vi "tag bus to outputs.vi"(9 "indices":T1, 11 "tag bus in":T3) -> (2 "data cluster":T2, 3 "tag bus out":T3)   [LabVIEW 2017, in "ActiveFrontEndModule runtime.lvclass"]
uses:
  ActiveFrontEndModule runtime.lvclass
  <vilib>/NI/Tag Bus/table/data table.ctl
  output user data.ctl
  configuration/output data indices.ctl
  <vilib>/NI/Tag Bus/table/data polymorphs/read one/read I32.vi
  <vilib>/NI/Tag Bus/table/data table.lvlib
  configuration/ActiveFrontEndModule configuration.lvclass
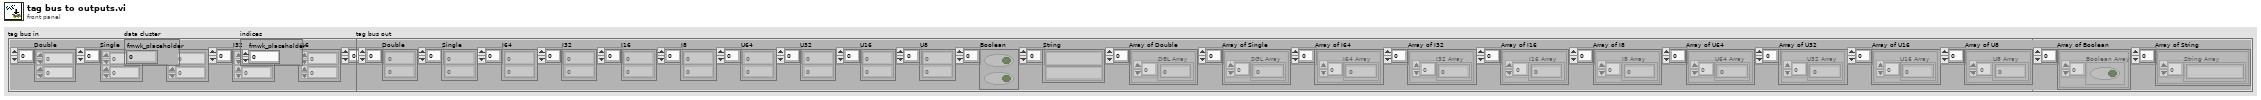
[diagram p1: front panel]
types:
  T1 = typedef "ActiveFrontEndModule configuration.lvclass/output data indices.ctl" = cluster{"fmwk_placeholder":i32}
  T2 = typedef "ActiveFrontEndModule runtime.lvclass/output user data.ctl" = cluster{"fmwk_placeholder":i32}
  T3 = typedef "tag bus.lvlib/data table.lvlib/data table.ctl" = cluster{"Double":dbl[], "Single":sgl[], "I64":i64[], "I32":i32[], "I16":i16[], "I8":i8[], "U64":u64[], "U32":u32[], "U16":u16[], "U8":u8[], "Boolean":bool[], "String":string[], "Array of Double":cluster{"DBL Array":dbl[]}[], "Array of Single":cluster{"SGL Array":sgl[]}[], "Array of I64":cluster{"I64 Array":i64[]}[], "Array of I32":cluster{"I32 Array":i32[]}[], "Array of I16":cluster{"I16 Array":i16[]}[], "Array of I8":cluster{"I8 Array":i8[]}[], "Array of U64":cluster{"U64 Array":u64[]}[], "Array of U32":cluster{"U32 Array":u32[]}[], "Array of U16":cluster{"U16 Array":u16[]}[], "Array of U8":cluster{"U8 Array":u8[]}[], "Array of Boolean":cluster{"Boolean Array":bool[]}[], "Array of String":cluster{"String Array":string[]}[]}
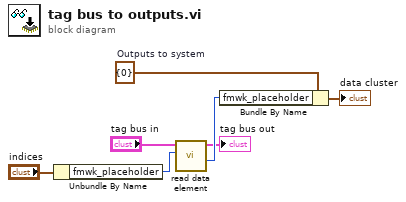
[diagram p0: block diagram]
diagram:
  w6 = T2 {"fmwk_placeholder"=0}  # Outputs to system
  n1 = Unbundle By Name("indices") -> ("fmwk_placeholder"=w2:i32)
  n2 = call-poly <vilib>:"read data element.vi"("index"=w2, "data table in"="tag bus in") -> ("value"=w3:i32, "data table out"=→"tag bus out":T3)  [unwired: 8 in]
  n3 = Bundle By Name(cluster=w6, "fmwk_placeholder"=w3) -> (→"data cluster":T2)
